vi "Read Parameter File.vi"(8 "error in (no error)":errorcluster, 11 "CD Parameter Manager in":refnum<class "CD Parameter Manager.lvclass">) -> (0 "error out":errorcluster, 3 "CD Parameter Manager out":refnum<class "CD Parameter Manager.lvclass">)   [LabVIEW 2019, in "CD Parameter Manager API.lvlib" / "CD Parameter Manager.lvclass"]
uses:
  CD Parameter Manager.lvclass
  CD Parameter Manager.lvclass/CD Parameter Manager.ctl
  Parameter Generic File/Parameter Generic File.lvclass
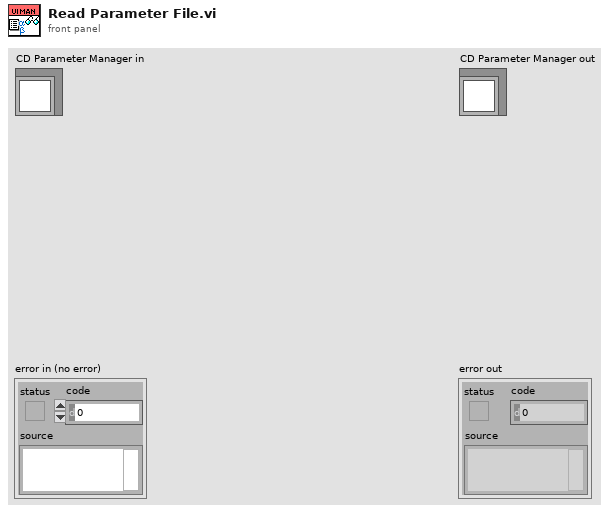
[diagram p1: front panel]
types:
  T1 = cluster{"Group name":string, "Controls":refnum<class "Parameter.lvclass">[]}[]
  T2 = cluster{"Group name":string, "Controls":refnum<class "Parameter.lvclass">[]}
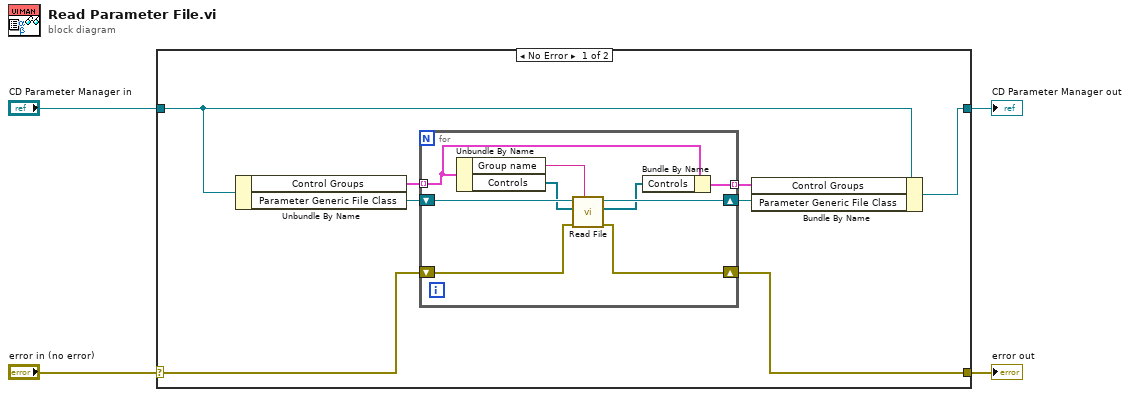
[diagram p0: block diagram]
diagram:
  n1 = case shown="No Error" "error in (no error)" {
    selector: "error in (no error)" -> [w11 w23]
    tunnel: [w10 w23] -> w3
    tunnel: [w8 w22] -> w1
    tunnel: "CD Parameter Manager in" -> [w9 w22]
    frame No Error {
      n2 = Unbundle By Name(w9) -> ("Control Groups"=w6:T1, "Parameter Generic File Class"=w12:refnum<class "Parameter Generic File.lvclass">)
      n3 = for {
        shift-right: [w18] -> w7
        shift-left: w12 -> [w21]
        shift-right: [w19] -> w10
        shift-left: w11 -> [w20]
        tunnel: w6 -> [w15] mode=indexing
        tunnel: [w13] -> w5 mode=indexing
        n4 = Unbundle By Name(w15) -> ("Group name"=w16:string, "Controls"=w17:refnum<class "Parameter.lvclass">[])
        n5 = call-dynamic "Read File.vi"("Section"=w16, "error in (no error)"=w20, "Parameters in"=w17, "Parameter Generic File in"=w21) -> ("error out"=w19:errorcluster, "Parameters out"=w14:refnum<class "Parameter.lvclass">[], "Parameter Generic File out"=w18:refnum<class "Parameter Generic File.lvclass">)  [unwired: 5 in]
        n6 = Bundle By Name(cluster=w15, "Controls"=w14) -> (w13:T2)
      }
      n7 = Bundle By Name(cluster=w9, "Control Groups"=w5, "Parameter Generic File Class"=w7) -> (w8:refnum<class "CD Parameter Manager.lvclass">)
    }
    frame Error {
    }
  }
  "error out" <- w3
  "CD Parameter Manager out" <- w1
